vi "MQTT_ConnAck_Read.vi"(8 "error in (no error)":errorcluster, 11 "connection ID":refnum<k5>) -> (0 "error out":errorcluster, 1 "QoS Level":T2, 2 "Connection Status":T1=enum."Connection refused: not authorized", 3 "connection ID out":refnum<k5>, 5 "MessageType":T3)   [LabVIEW 2017, in "MQTT_Functions.lvlib"]
doc: "This VI processes the connection acknowledge message from the server.\n\n© 2015 - daq.io, LLC - Peter Adelhardt"
uses:
  MQTT_Functions.lvlib
  Controls/MessageType.ctl
  Controls/QoS.ctl
  Controls/Connection_Return_Codes.ctl
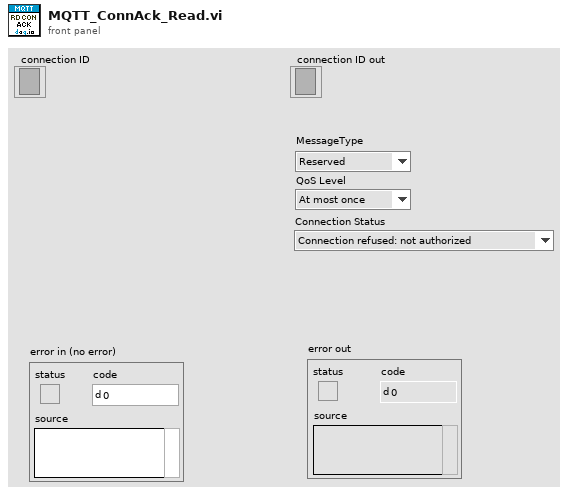
[diagram p1: front panel]
types:
  T1 = typedef "MQTT_Functions.lvlib/Connection_Return_Codes.ctl" = enum16{"Connection accepted", "Connection refused: unacceptable protocol version", "Connection refused: identifier rejected", "Connection refused: Server unavailable", "Connection refused: bad user name or password", "Connection refused: not authorized"}
  T2 = typedef "MQTT_Functions.lvlib/QoS.ctl" = enum8{"At most once", "At least once", "Exactly once", "Reserved"}
  T3 = typedef "MQTT_Functions.lvlib/MessageType.ctl" = enum32{"Reserved", "CONNECT", "CONNACK", "PUBLISH", "PUBACK", "PUBREC", "PUBREL", "PUBCOMP", "SUBSCRIBE", "SUBACK", "UNSUBSCRIBE", "UNSUBACK", "PINGREQ", "PINGRESP", "DISCONNECT", "Reserved2"}
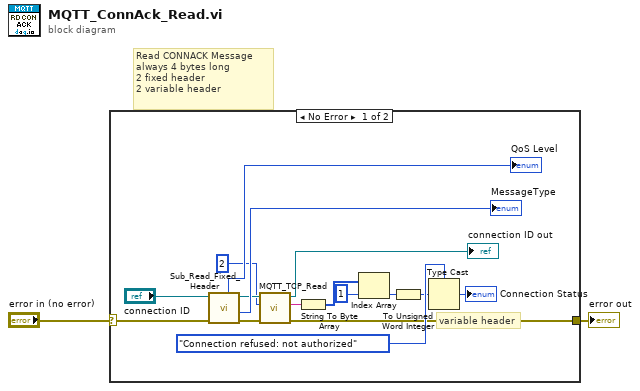
[diagram p0: block diagram]
diagram:
  # "Read CONNACK Message\nalways 4 bytes long\n2 fixed header\n2 variable header"
  n1 = case shown="No Error" "error in (no error)" {
    selector: "error in (no error)" -> [w16 w19]
    tunnel: [w7 w19] -> w1
    frame No Error {
      # "variable header"
      n2 = call "Sub_Read_Fixed_Header.vi"("error in (no error)"=w16, "connection ID"="connection ID") -> ("error out"=w8:errorcluster, "MessageType"=→"MessageType":T3, "connection ID out"=w10:refnum<k5>, "QoS Level"=→"QoS Level":T2)  [unwired: 3 in, 3 out]
      n3 = call "MQTT_TCP_Read.vi"("error in (no error)"=w8, "bytes to read"=2, "connection ID"=w10) -> ("error out"=w7:errorcluster, "data out"=w5:string, "connection ID out"=→"connection ID out":refnum<k5>)  [unwired: 6 in]
      n4 = String To Byte Array(string=w5) -> (unsigned byte array=w4:u8[])
      n5 = Index Array(array=w4, index=1) -> (element=w18:u8)
      n6 = To Unsigned Word Integer(number=w18) -> (unsigned 16bit integer=w3:u16)
      n7 = Type Cast(type=Connection_Return_Codes."Connection refused: not authorized" ("Conn Return Code"), x=w3) -> (*(type *) &x=→"Connection Status":T1)
    }
    frame Error {
    }
  }
  "error out" <- w1
